vi "StartByteDecoder.vi"(0 "byte1":string="Ò") -> (1 "Byte Start ?":bool)   [LabVIEW 2010]
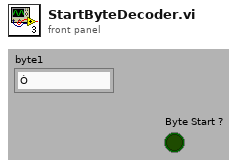
[diagram p1: front panel]
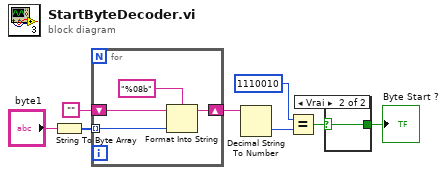
[diagram p0: block diagram]
diagram:
  n1 = String To Byte Array(string="byte1") -> (unsigned byte array=w3:u8[])
  n2 = for {
    tunnel: w3 -> [w12] mode=indexing
    shift-right: [w10] -> w5
    shift-left: "" -> [w11]
    n3 = Format Into String(format string="%08b" ("chaîne de format"), initial string=w11, w12) -> (resulting string=w10:string)  [unwired: 1 in, 1 out]
  }
  n4 = Decimal String To Number(string=w5) -> (number=w1:i32)  [unwired: 2 in, 1 out]
  n5 = Equal?(x=1110010, y=w1) -> (x = y?=w7:bool)
  n6 = case shown="Vrai" w7 {
    selector: w7 -> [w13 w14]
    tunnel: [w13 w14] -> w8
    frame False {
    }
    frame True {
    }
  }
  "Byte Start ?" <- w8
